vi "Extraction - Calculations.vi"(4 "Device":T1, 6 "Model":enum16{"pi", "tee"}(ring), 7 "2-port?":bool=TRUE, 8 "Freq for nominal C (MHz)":dbl=100.0, 9 "Y/Z-parameters":cdb[][](array[numeric]), 10 "Frequencies (Hz) in":dbl[](array[numeric]), 11 "S-parameters":cdb[][](array[numeric])) -> (0 "Heading":string[](array[string])=["Frequency (MHz)", "Capacitance (pF)", "Resistance (Ohm)", "Q", "Cshunt1 (pF)", "Cshunt2 (pF)", "SRF (MHz)"], 1 "index file values":dbl[](array[numeric]), 2 "index file heading":string[](array[string]), 3 "Frequency,C, R, Q/-IL, L, Cshunt1/2, Rshunt1/2, Lshunt1/2, SRF":dbl[][](array[numeric]), 5 "Graphs":T2)   [LabVIEW 2020]
panel:
  out "SRF (MHz)":dbl[](array[numeric])
  out "L":cluster{"Frequencies (Hz) in":dbl[], dbl[]}[](graph)
  out "S-para (mag)":dbl[][](array[numeric])
  out "Q":cluster{"Frequencies (Hz)":dbl[], dbl[]}(graph)
  out "R":cluster{"Frequencies (Hz)":dbl[], dbl[]}(graph)
  out "Capa":cluster{"Frequencies (Hz) in":dbl[], dbl[]}[](graph)
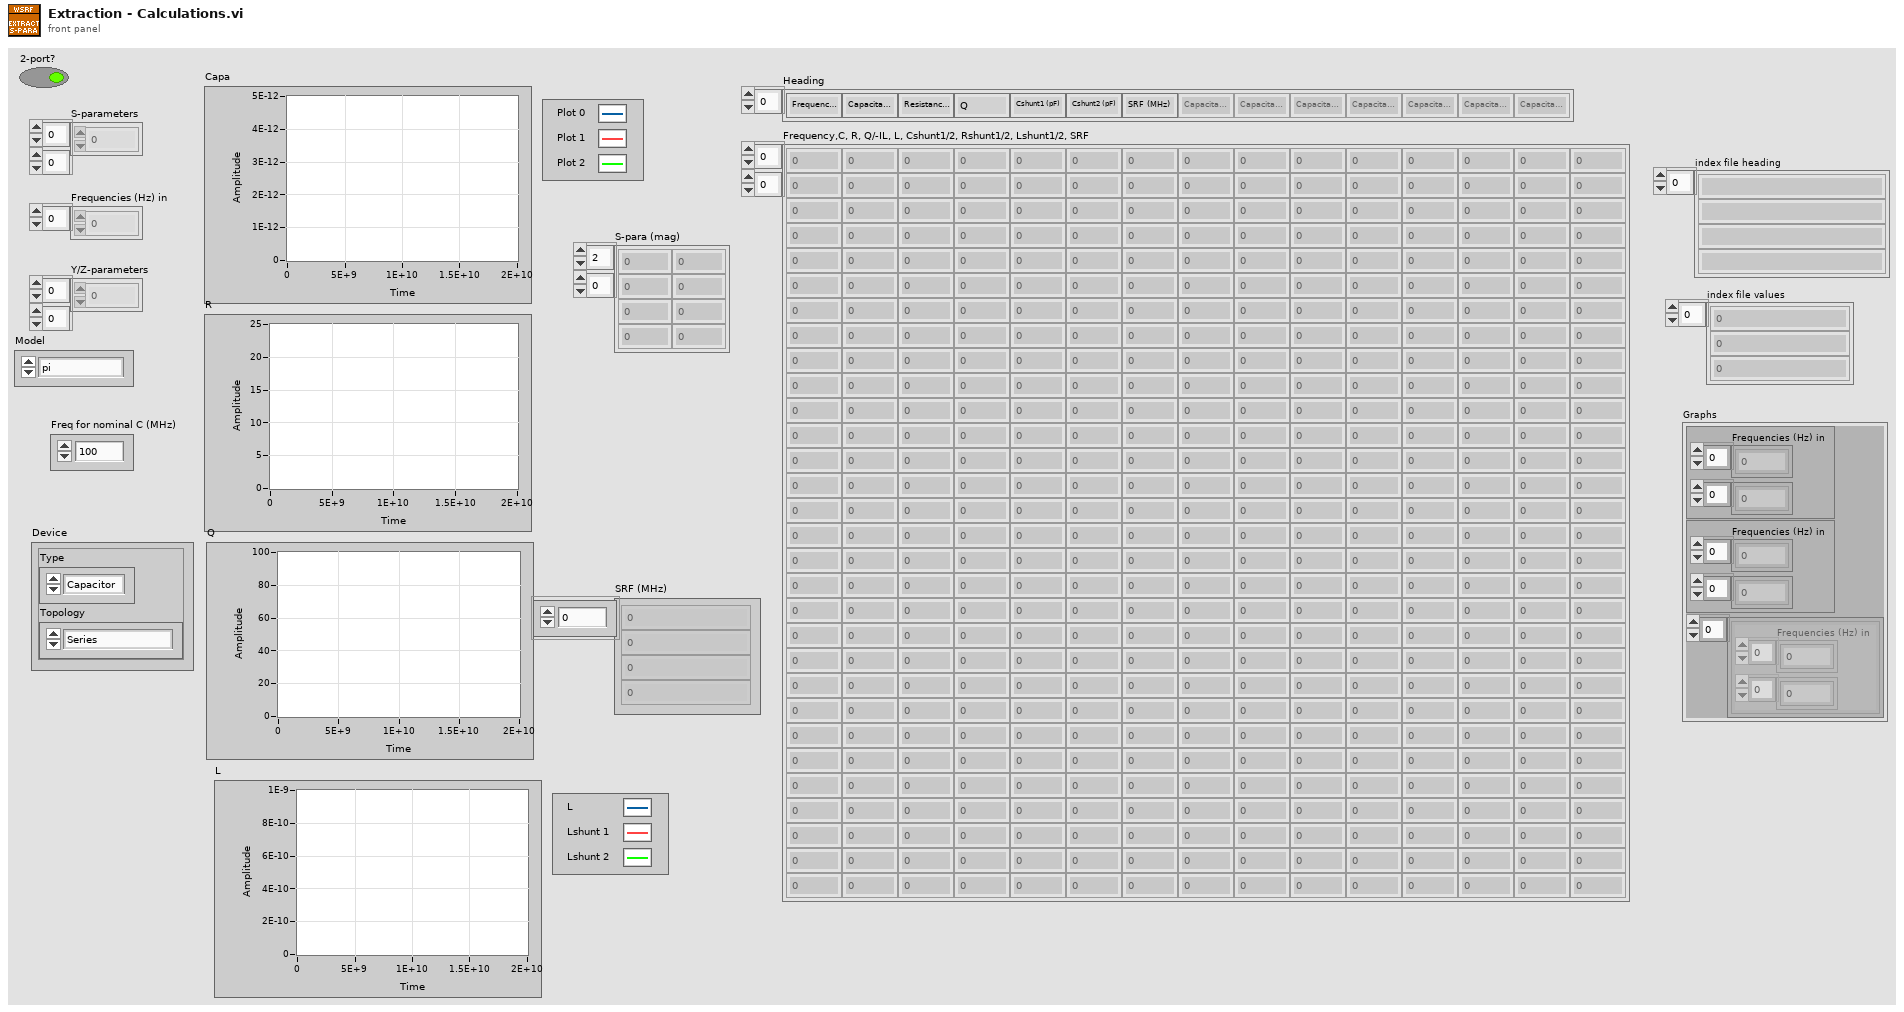
[diagram p1: front panel]
types:
  T1 = cluster{"Type":enum16{"Capacitor", "Switch"}, "Topology":enum16{"Series", "Parallel"}}
  T2 = cluster{cluster{"Frequencies (Hz) in":dbl[], dbl[]}, cluster{"Frequencies (Hz) in":dbl[], dbl[]}, cluster{"Frequencies (Hz) in":dbl[], dbl[]}[]}
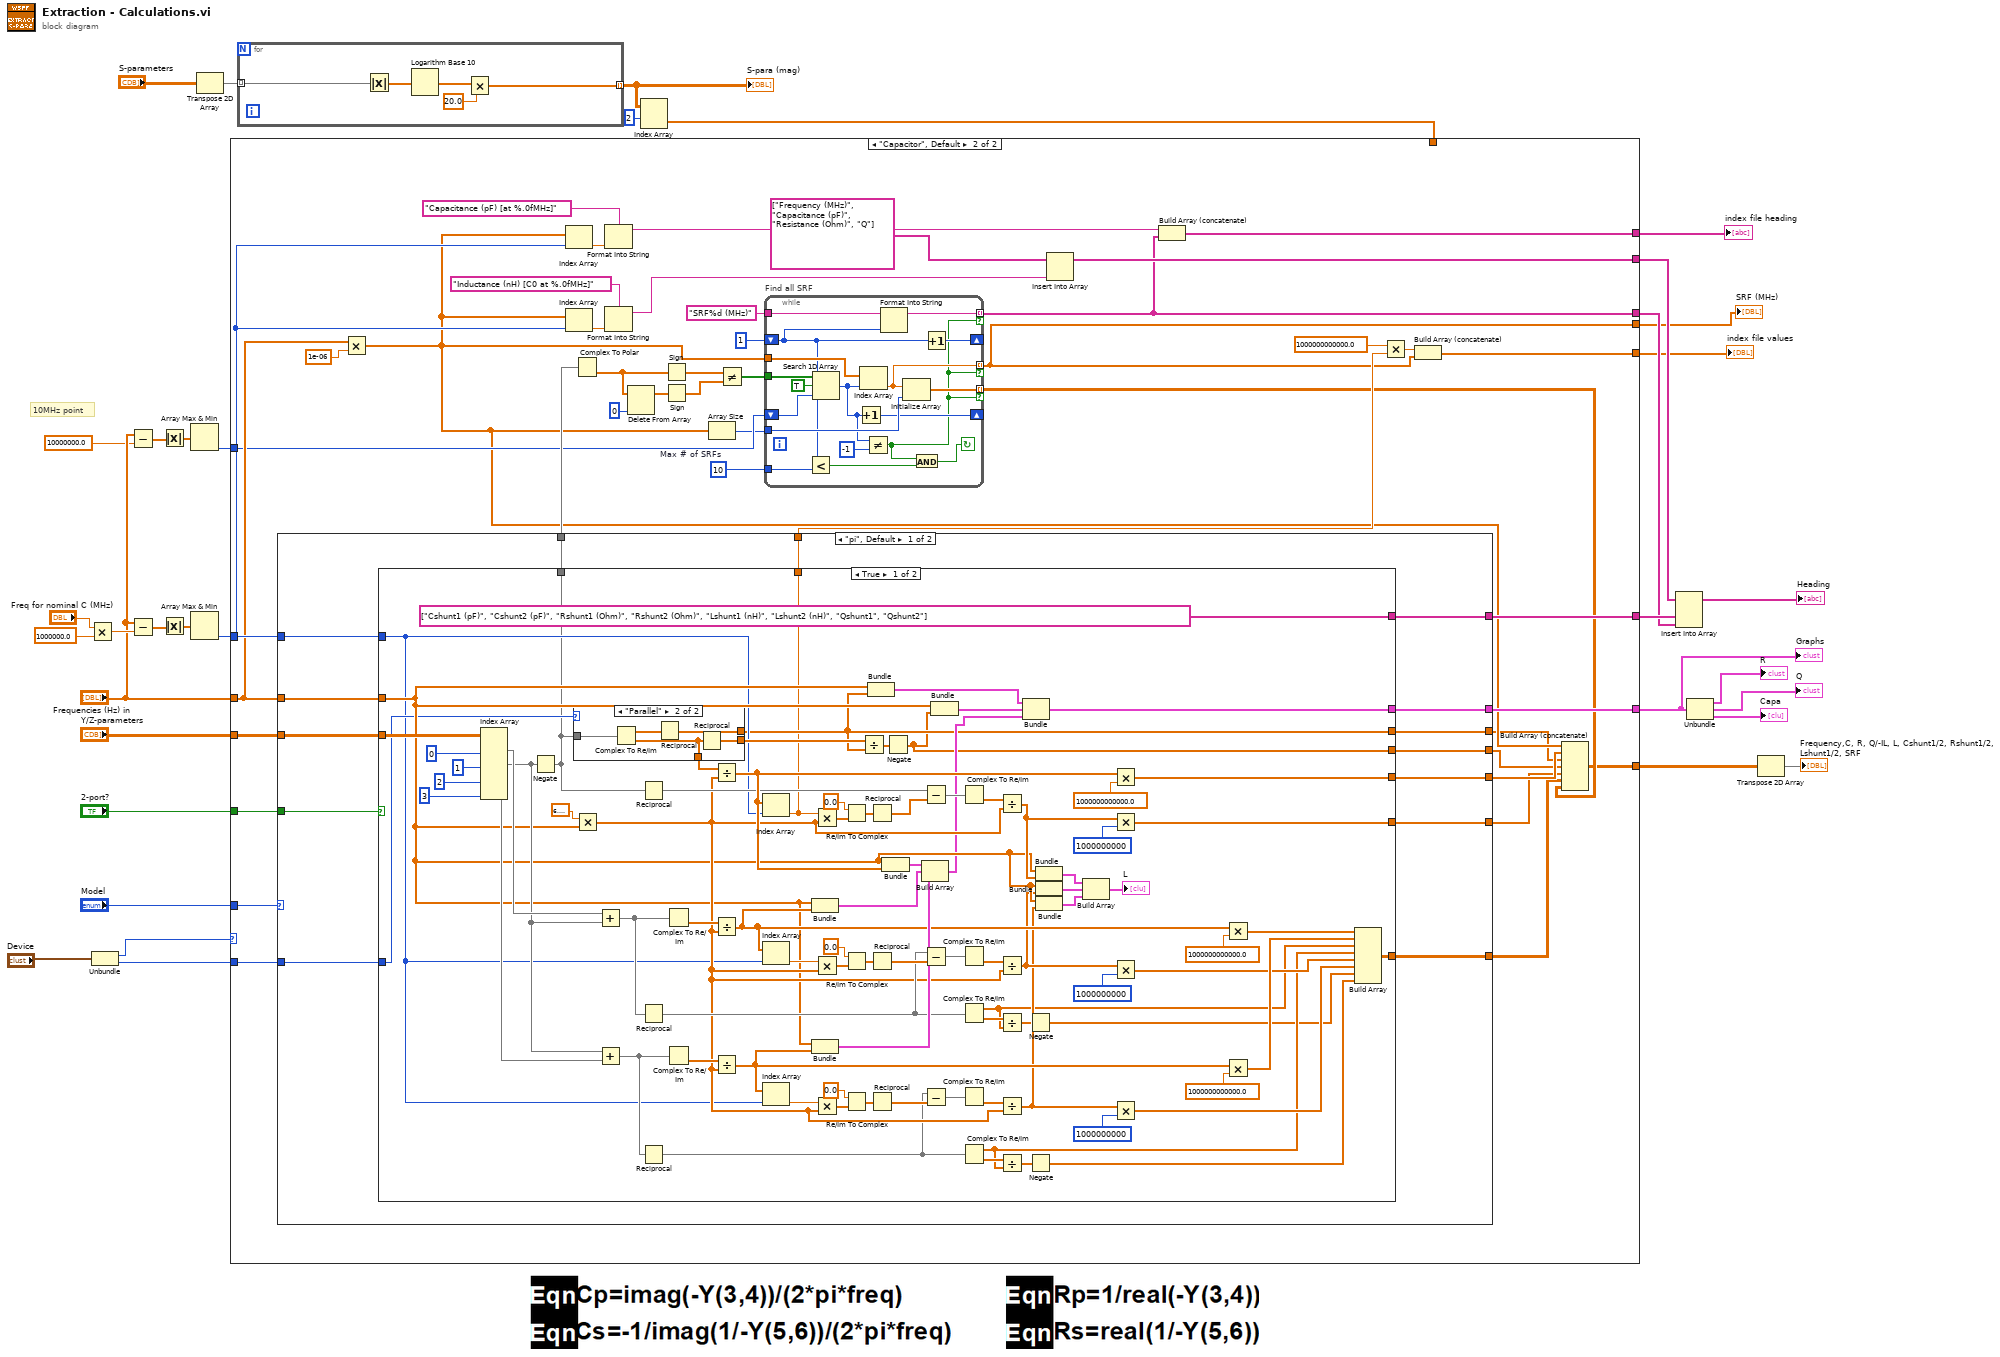
[diagram p0: block diagram]
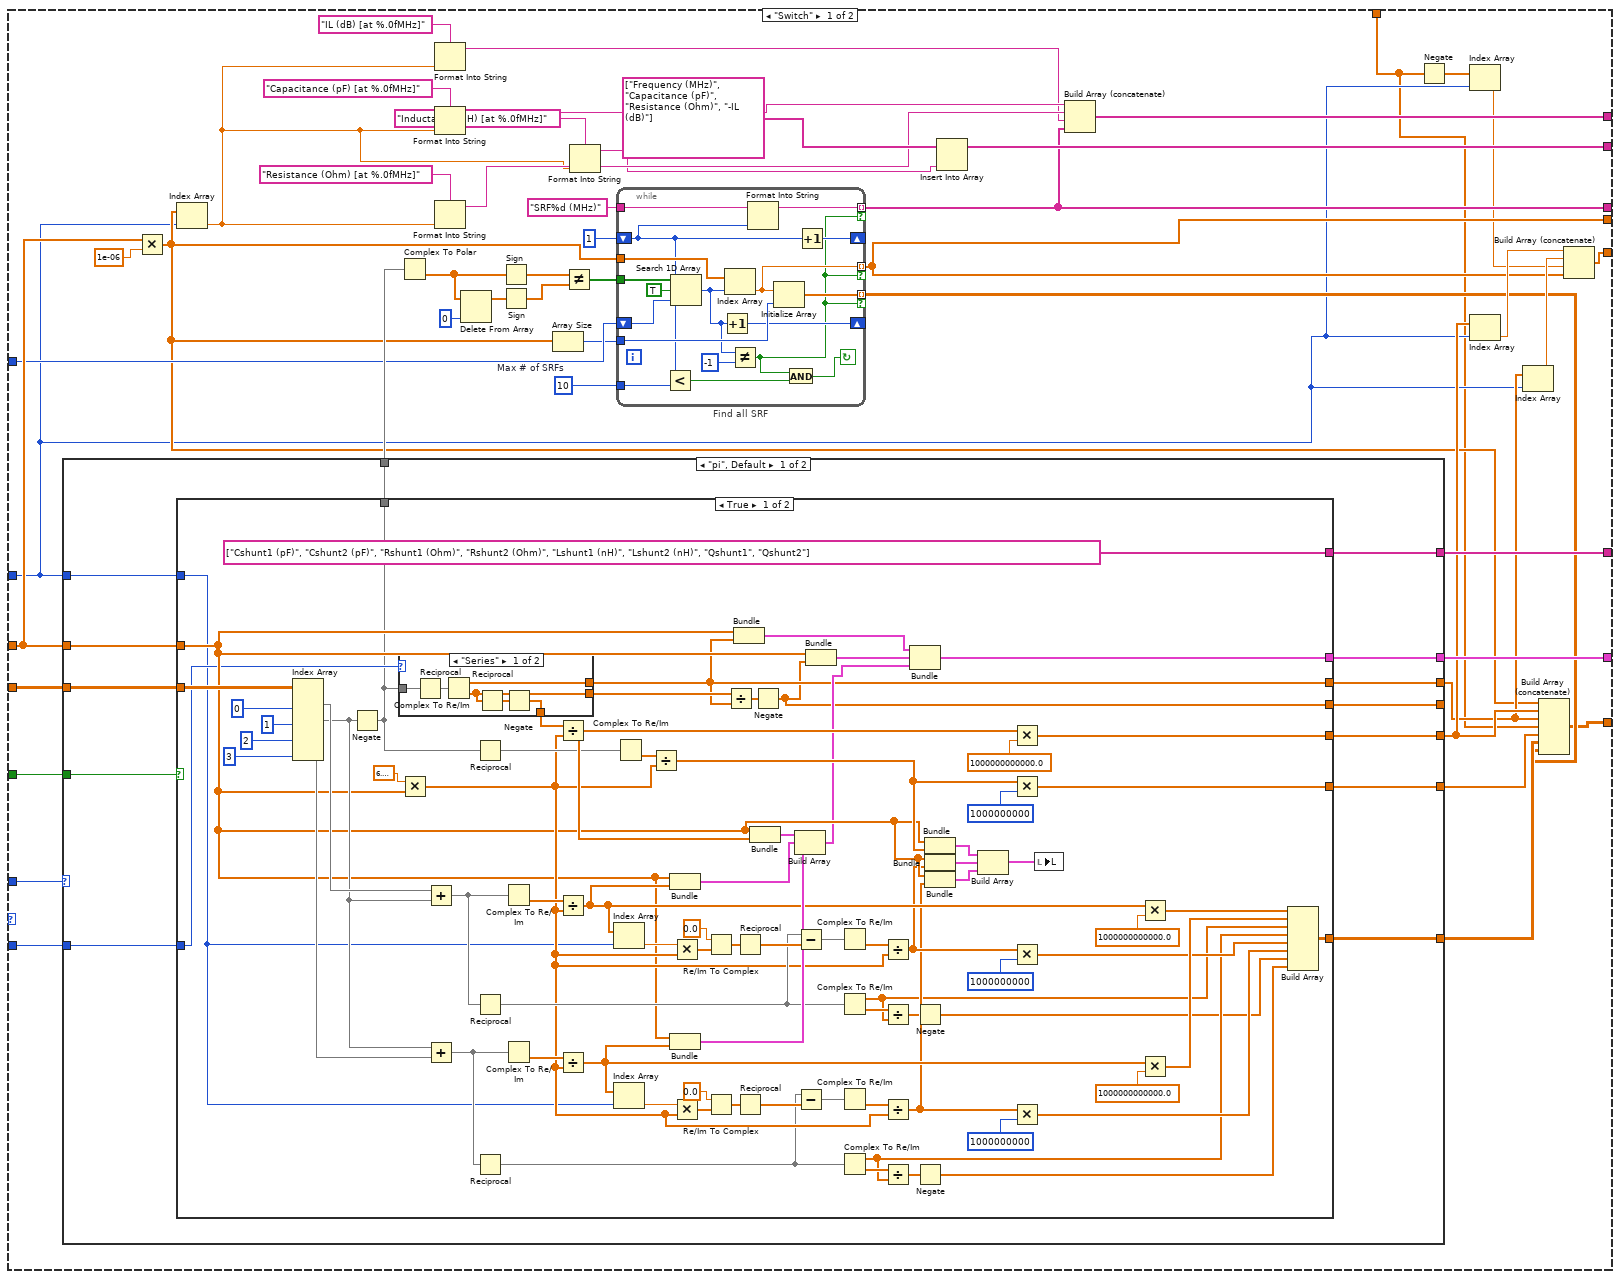
[diagram p2: hidden frame]
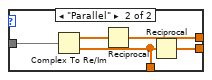
[diagram p3: hidden frame]
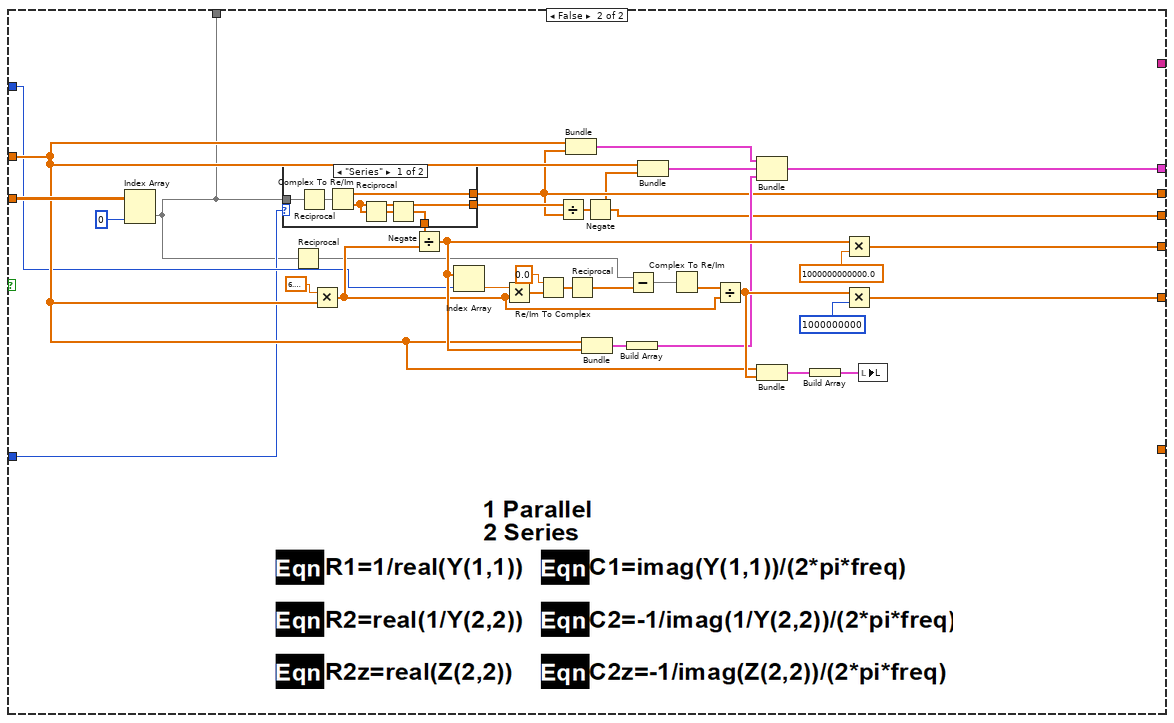
[diagram p4: hidden frame]
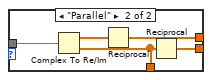
[diagram p5: hidden frame]
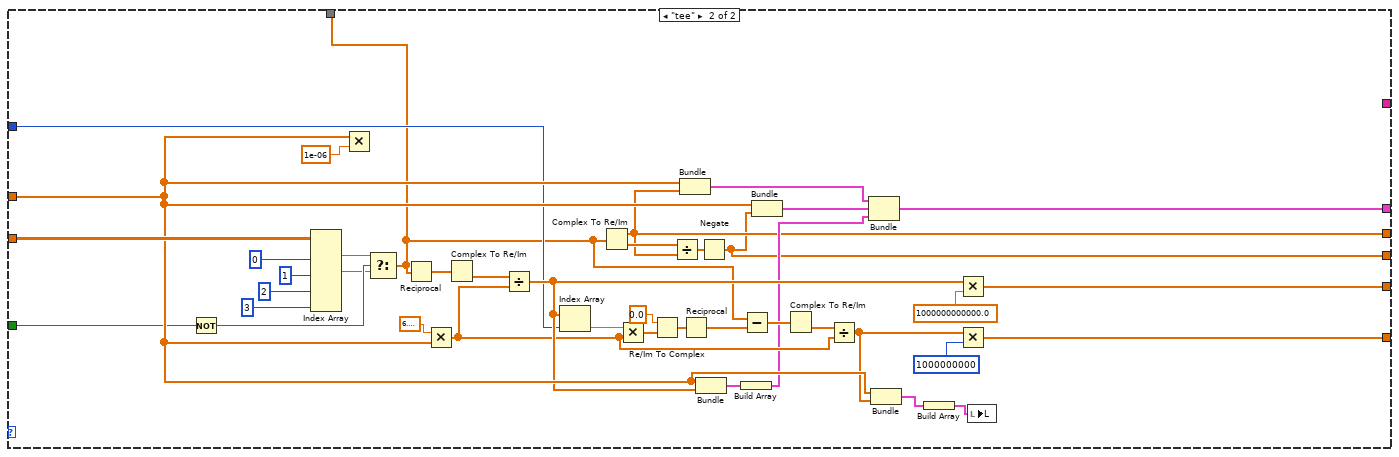
[diagram p6: hidden frame]
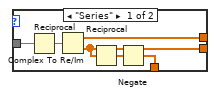
[diagram p7: hidden frame]
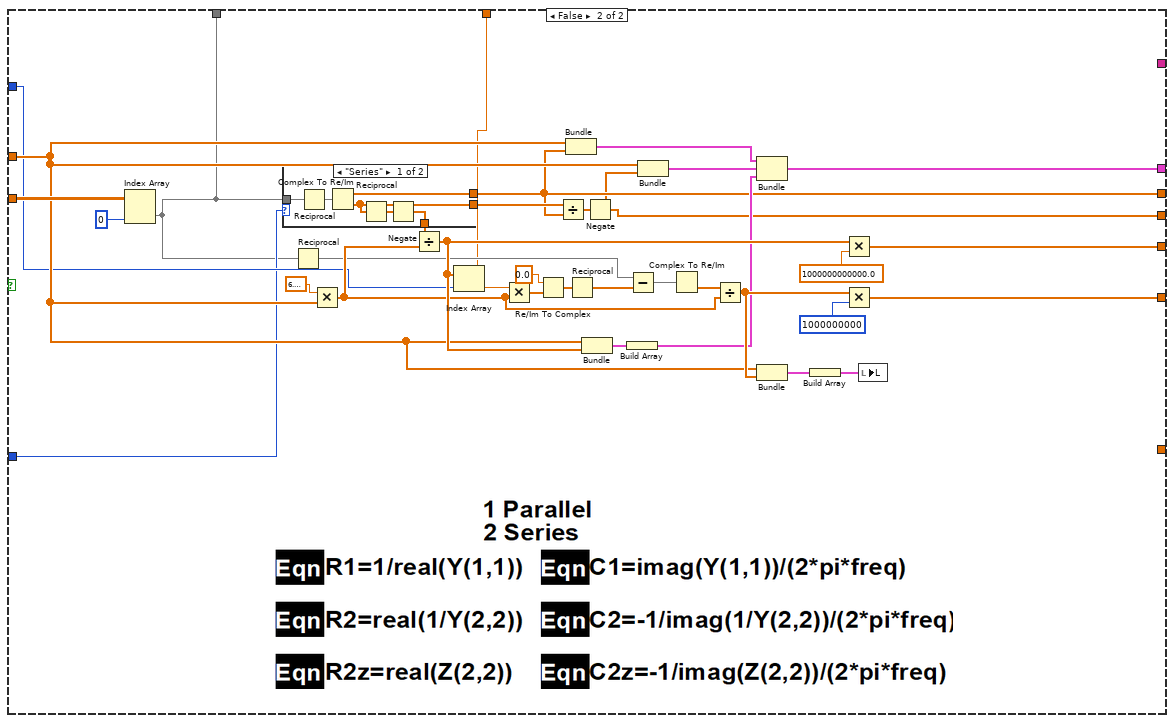
[diagram p8: hidden frame]
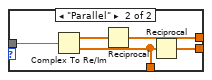
[diagram p9: hidden frame]
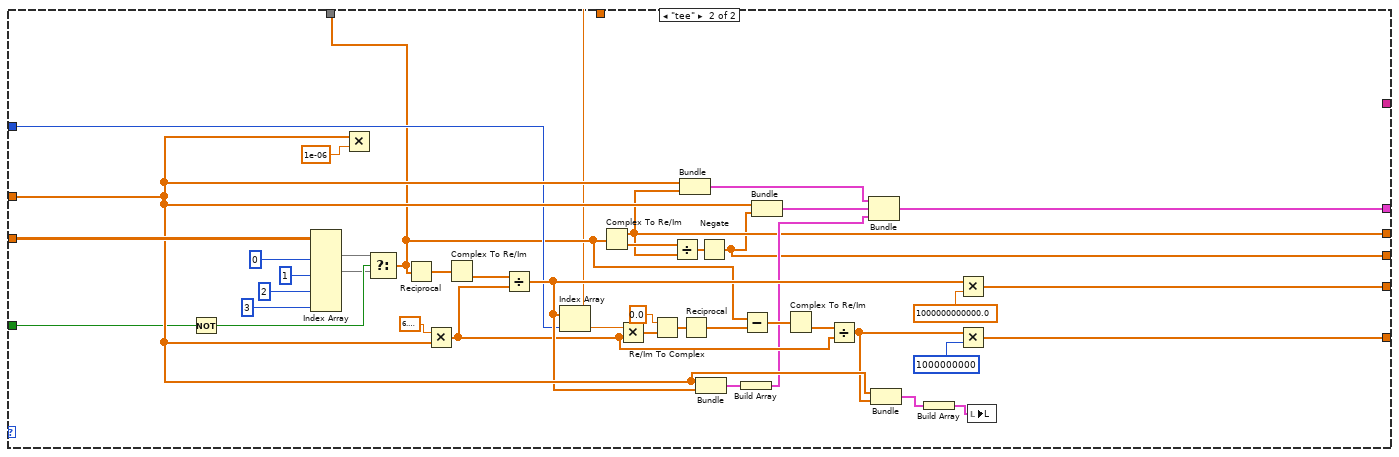
[diagram p10: hidden frame]
diagram:
  # "10MHz point"
  n1 = Multiply(x="Freq for nominal C (MHz)", y=1000000.0 ("Frequency (Hz)")) -> (x*y=w27:dbl)
  n2 = Unbundle("Device") -> ("Type"=w8:enum16{"Capacitor", "Switch"}, "Topology"=w9:enum16{"Series", "Parallel"})
  n3 = Subtract(x="Frequencies (Hz) in", y=10000000.0 ("Frequency (Hz)")) -> (x-y=w17:dbl[])
  n4 = Subtract(x="Frequencies (Hz) in", y=w27) -> (x-y=w26:dbl[])
  n5 = Absolute Value(x=w17) -> (abs(x)=w16:dbl[])
  n6 = Absolute Value(x=w26) -> (abs(x)=w25:dbl[])
  n7 = Array Max & Min(array=w16) -> (min index (indices)=w15:i32)  [unwired: 3 out]
  n8 = Array Max & Min(array=w25) -> (min index (indices)=w20:i32)  [unwired: 3 out]
  n9 = Transpose 2D Array(2D array="S-parameters") -> (transposed array=w32:cdb[][])
  n10 = for {
    tunnel: w32 -> [w37] mode=indexing
    tunnel: [w36] -> w3 mode=indexing
    n11 = Absolute Value(x=w37) -> (abs(x)=w38:dbl[])
    n12 = Logarithm Base 10(1:w38) -> (0:w39:dbl[])
    n13 = Multiply(x=w39, y=20.0) -> (x*y=w36:dbl[])
  }
  "S-para (mag)" <- w3
  n14 = Index Array(array=w3, index (row)=2) -> (element=w1:dbl[])  [unwired: 1 in]
  n15 = case shown="\"Capacitor\", Default" w8 {
    tunnel: "Y/Z-parameters" -> [w88 w340]
    tunnel: "2-port?" -> [w87 w339]
    tunnel: "Model" -> [w86 w338]
    tunnel: [w85 w337] -> w21
    tunnel: w20 -> [w47 w330]
    tunnel: "Frequencies (Hz) in" -> [w72 w317]
    tunnel: w15 -> [w71 w316]
    tunnel: [w67 w312] -> w13
    tunnel: [w66 w311] -> w12
    tunnel: [w65 w310] -> w11
    tunnel: w9 -> [w63 w308]
    tunnel: [w58 w307] -> w7
    tunnel: [w57 w306] -> w6
    tunnel: [w56 w305] -> w5
    tunnel: [w53 w298] -> w4
    tunnel: w1 -> [w42 _]
    frame "Switch" {
      w64 = 10  # Max # of SRFs
      n16 = case shown="\"pi\", Default" w86 {
        tunnel: w88 -> [w119 w296]
        tunnel: w72 -> [w114 w295]
        tunnel: w87 -> [w118 w294]
        tunnel: w47 -> [w115 w266]
        tunnel: w63 -> [w117 _]
        tunnel: [w116 w262] -> w85
        tunnel: [w110 w261] -> w74
        tunnel: [w107 w259] -> w61
        tunnel: [w113 w258] -> w51
        tunnel: [w112 w257] -> _
        tunnel: [w108 w256] -> w62
        tunnel: [w111 _] -> w55
        tunnel: [w109 _] -> w67
        frame "pi", Default {
          n17 = case shown="True" w118 {
            tunnel: [w198 _] -> w111
            tunnel: w119 -> [w193 w240]
            tunnel: w114 -> [w145 w226]
            tunnel: w115 -> [w122 w224]
            tunnel: w117 -> [w132 w223]
            tunnel: [w128 w217] -> w116
            tunnel: [w121 w216] -> w107
            tunnel: [w127 w215] -> w113
            tunnel: [w126 w214] -> w112
            tunnel: [w123 w213] -> w108
            tunnel: [w125 w211] -> w110
            tunnel: [string[] ["Cshunt1 (pF)", "Cshunt2 (pF)", "Rshunt1 (Ohm)", "Rshunt2 (Ohm)", "Lshunt1 (nH)", "Lshunt2 (nH)", "Qshunt1", "Qshunt2"] ("Heading") _] -> w109
            frame True {
              n18 = Index Array(array=w193, index (col) #1=0 ("disabled index (col)"), index (col) #2=1 ("disabled index (col)"), index (col) #3=2 ("index (col)"), index (col) #4=3 ("index (col)")) -> (element #1=w190:cdb[], element #2=w187:cdb[], element #4=w186:cdb[])  [unwired: 4 in, 1 out]
              n19 = Negate(x=w187) -> (-x=w125:cdb[])
              n20 = case shown="\"Series\"" w132 {
                tunnel: [w205 w208] -> w127
                tunnel: [w202 w207] -> w133
                tunnel: w125 -> [w204 w210]
                tunnel: [w200 w206] -> w134
                frame "Series" {
                  n21 = Reciprocal(x=w204) -> (1/x=w203:cdb[])
                  n22 = Complex To Re/Im(x + iy=w203) -> (x=w205:dbl[], y=w202:dbl[])
                  n23 = Reciprocal(x=w202) -> (1/x=w201:dbl[])
                  n24 = Negate(x=w201) -> (-x=w200:dbl[])
                }
                frame "Parallel" {
                  n25 = Complex To Re/Im(x + iy=w210) -> (x=w209:dbl[], y=w206:dbl[])
                  n26 = Reciprocal(x=w209) -> (1/x=w208:dbl[])
                  n27 = Reciprocal(x=w206) -> (1/x=w207:dbl[])
                }
              }
              n28 = Multiply(x=6.283185307179586, y=w145) -> (x*y=w155:dbl[])
              n29 = Add(x=w190, y=w187) -> (x+y=w175:cdb[])
              n30 = Add(x=w187, y=w186) -> (x+y=w174:cdb[])
              n31 = Reciprocal(x=w125) -> (1/x=w167:cdb[])
              n32 = Reciprocal(x=w175) -> (1/x=w156:cdb[])
              n33 = Reciprocal(x=w174) -> (1/x=w150:cdb[])
              n34 = Complex To Re/Im(x + iy=w175) -> (y=w189:dbl[])  [unwired: 1 out]
              n35 = Complex To Re/Im(x + iy=w174) -> (y=w188:dbl[])  [unwired: 1 out]
              n36 = Divide(x=w134, y=w155) -> (x/y=w178:dbl[])
              n37 = Divide(x=w189, y=w155) -> (x/y=w176:dbl[])
              n38 = Divide(x=w188, y=w155) -> (x/y=w177:dbl[])
              n39 = Index Array(array=w176, index=w122) -> (element=w173:dbl)
              n40 = Index Array(array=w177, index=w122) -> (element=w172:dbl)
              n41 = Complex To Re/Im(x + iy=w167) -> (y=w166:dbl[])  [unwired: 1 out]
              n42 = Divide(x=w166, y=w155) -> (x/y=w148:dbl[])
              n43 = Bundle("Frequencies (Hz) in"=w145, w176) -> (w182:cluster{"Frequencies (Hz) in":dbl[], dbl[]})  [unwired: 1 in]
              n44 = Bundle("Frequencies (Hz) in"=w145, w177) -> (w181:cluster{"Frequencies (Hz) in":dbl[], dbl[]})  [unwired: 1 in]
              n45 = Multiply(x=w173, y=w155) -> (x*y=w171:dbl[])
              n46 = Multiply(x=w172, y=w155) -> (x*y=w170:dbl[])
              n47 = Re/Im To Complex(1:w171, 2:0.0) -> (0:w161:cdb[])
              n48 = Re/Im To Complex(1:w170, 2:0.0) -> (0:w157:cdb[])
              n49 = Divide(x=w133, y=w127) -> (x/y=w197:dbl[])
              n50 = Bundle("Frequencies (Hz) in"=w145, w127) -> (w129:cluster{"Frequencies (Hz) in":dbl[], dbl[]})  [unwired: 1 in]
              n51 = Reciprocal(x=w161) -> (1/x=w162:cdb[])
              n52 = Reciprocal(x=w157) -> (1/x=w160:cdb[])
              n53 = Bundle("Frequencies (Hz) in"=w145, w178) -> (w180:cluster{"Frequencies (Hz) in":dbl[], dbl[]})  [unwired: 1 in]
              n54 = Negate(x=w197) -> (-x=w126:dbl[])
              n55 = Build Array(w180, w182, w181) -> (w131:cluster{"Frequencies (Hz) in":dbl[], dbl[]}[])
              n56 = Subtract(x=w156, y=w162) -> (x-y=w163:cdb[])
              n57 = Subtract(x=w150, y=w160) -> (x-y=w159:cdb[])
              n58 = Bundle("Frequencies (Hz) in"=w145, w126) -> (w130:cluster{"Frequencies (Hz) in":dbl[], dbl[]})  [unwired: 1 in]
              n59 = Complex To Re/Im(x + iy=w163) -> (y=w164:dbl[])  [unwired: 1 out]
              n60 = Complex To Re/Im(x + iy=w156) -> (x=w136:dbl[], y=w137:dbl[])
              n61 = Complex To Re/Im(x + iy=w159) -> (y=w158:dbl[])  [unwired: 1 out]
              n62 = Complex To Re/Im(x + iy=w150) -> (x=w141:dbl[], y=w142:dbl[])
              n63 = Divide(x=w164, y=w155) -> (x/y=w144:dbl[])
              n64 = Divide(x=w137, y=w136) -> (x/y=w138:dbl[])
              n65 = Divide(x=w158, y=w155) -> (x/y=w143:dbl[])
              n66 = Divide(x=w142, y=w141) -> (x/y=w140:dbl[])
              n67 = Bundle(w129, w130, w131) -> (w128:T2)  [unwired: 1 in]
              n68 = Negate(x=w138) -> (-x=w135:dbl[])
              n69 = Negate(x=w140) -> (-x=w139:dbl[])
              n70 = Bundle("Frequencies (Hz) in"=w145, w148) -> (w149:cluster{"Frequencies (Hz) in":dbl[], dbl[]})  [unwired: 1 in]
              n71 = Bundle("Frequencies (Hz) in"=w145, w144) -> (w147:cluster{"Frequencies (Hz) in":dbl[], dbl[]})  [unwired: 1 in]
              n72 = Bundle("Frequencies (Hz) in"=w145, w143) -> (w146:cluster{"Frequencies (Hz) in":dbl[], dbl[]})  [unwired: 1 in]
              n73 = Build Array(w149, w147, w146) -> (w120:cluster{"Frequencies (Hz) in":dbl[], dbl[]}[])
              n74 = Multiply(x=w178, y=1000000000000.0 ("Frequency (Hz)")) -> (x*y=w121:dbl[])
              n75 = Multiply(x=w148, y=1000000000 ("Frequency (Hz)")) -> (x*y=w123:dbl[])
              n76 = Multiply(x=w144, y=1000000000 ("Frequency (Hz)")) -> (x*y=w152:dbl[])
              n77 = Multiply(x=w143, y=1000000000 ("Frequency (Hz)")) -> (x*y=w151:dbl[])
              n78 = local write "L"(w120) -> ()
              n79 = Multiply(x=w176, y=1000000000000.0 ("Frequency (Hz)")) -> (x*y=w179:dbl[])
              n80 = Multiply(x=w177, y=1000000000000.0 ("Frequency (Hz)")) -> (x*y=w183:dbl[])
              n81 = Build Array(w179, w183, w136, w141, w152, w151, w135, w139) -> (w198:dbl[][])
            }
            frame False {
              n82 = Index Array(array=w240, index (col)=0 ("disabled index (col)")) -> (element=w211:cdb[])  [unwired: 1 in]
              n83 = case shown="\"Series\"" w223 {
                tunnel: [w250 w253] -> w215
                tunnel: [w247 w252] -> w243
                tunnel: w211 -> [w249 w255]
                tunnel: [w245 w251] -> w221
                frame "Series" {
                  n84 = Reciprocal(x=w249) -> (1/x=w248:cdb[])
                  n85 = Complex To Re/Im(x + iy=w248) -> (x=w250:dbl[], y=w247:dbl[])
                  n86 = Reciprocal(x=w247) -> (1/x=w246:dbl[])
                  n87 = Negate(x=w246) -> (-x=w245:dbl[])
                }
                frame "Parallel" {
                  n88 = Complex To Re/Im(x + iy=w255) -> (x=w254:dbl[], y=w251:dbl[])
                  n89 = Reciprocal(x=w254) -> (1/x=w253:dbl[])
                  n90 = Reciprocal(x=w251) -> (1/x=w252:dbl[])
                }
              }
              n91 = Reciprocal(x=w211) -> (1/x=w222:cdb[])
              n92 = Multiply(x=6.283185307179586, y=w226) -> (x*y=w229:dbl[])
              n93 = Divide(x=w221, y=w229) -> (x/y=w237:dbl[])
              n94 = Index Array(array=w237, index=w224) -> (element=w212:dbl)
              n95 = Multiply(x=w212, y=w229) -> (x*y=w236:dbl[])
              n96 = Re/Im To Complex(1:w236, 2:0.0) -> (0:w234:cdb[])
              n97 = Divide(x=w243, y=w215) -> (x/y=w244:dbl[])
              n98 = Bundle("Frequencies (Hz) in"=w226, w215) -> (w220:cluster{"Frequencies (Hz) in":dbl[], dbl[]})  [unwired: 1 in]
              n99 = Reciprocal(x=w234) -> (1/x=w233:cdb[])
              n100 = Bundle("Frequencies (Hz) in"=w226, w237) -> (w238:cluster{"Frequencies (Hz) in":dbl[], dbl[]})  [unwired: 1 in]
              n101 = Negate(x=w244) -> (-x=w214:dbl[])
              n102 = Build Array(w238) -> (w218:cluster{"Frequencies (Hz) in":dbl[], dbl[]}[])
              n103 = Subtract(x=w222, y=w233) -> (x-y=w232:cdb[])
              n104 = Bundle("Frequencies (Hz) in"=w226, w214) -> (w219:cluster{"Frequencies (Hz) in":dbl[], dbl[]})  [unwired: 1 in]
              n105 = Complex To Re/Im(x + iy=w232) -> (y=w231:dbl[])  [unwired: 1 out]
              n106 = Divide(x=w231, y=w229) -> (x/y=w227:dbl[])
              n107 = Bundle(w220, w219, w218) -> (w217:T2)  [unwired: 1 in]
              n108 = Bundle("Frequencies (Hz) in"=w226, w227) -> (w228:cluster{"Frequencies (Hz) in":dbl[], dbl[]})  [unwired: 1 in]
              n109 = Build Array(w228) -> (w225:cluster{"Frequencies (Hz) in":dbl[], dbl[]}[])
              n110 = Multiply(x=w237, y=1000000000000.0 ("Frequency (Hz)")) -> (x*y=w216:dbl[])
              n111 = Multiply(x=w227, y=1000000000 ("Frequency (Hz)")) -> (x*y=w213:dbl[])
              n112 = local write "L"(w225) -> ()
            }
          }
        }
        frame "tee" {
          n113 = Not(x=w294) -> (.not. x?=w269:bool)
          n114 = Index Array(array=w296, index (col) #1=0 ("disabled index (col)"), index (col) #2=1 ("disabled index (col)"), index (col) #3=2 ("index (col)"), index (col) #4=3 ("index (col)")) -> (element #1=w268:cdb[], element #2=w267:cdb[])  [unwired: 4 in, 2 out]
          n115 = Multiply(x=w295, y=1e-06 ("Frequency (Hz)")) -> ()  [unwired: 1 out]
          n116 = Select(t=w268, s=w269, f=w267) -> (s? t:f=w261:cdb[])
          n117 = Reciprocal(x=w261) -> (1/x=w270:cdb[])
          n118 = Multiply(x=6.283185307179586, y=w295) -> (x*y=w274:dbl[])
          n119 = Complex To Re/Im(x + iy=w270) -> (y=w287:dbl[])  [unwired: 1 out]
          n120 = Divide(x=w287, y=w274) -> (x/y=w282:dbl[])
          n121 = Index Array(array=w282, index=w266) -> (element=w260:dbl)
          n122 = Complex To Re/Im(x + iy=w261) -> (x=w258:dbl[], y=w291:dbl[])
          n123 = Multiply(x=w260, y=w274) -> (x*y=w281:dbl[])
          n124 = Re/Im To Complex(1:w281, 2:0.0) -> (0:w279:cdb[])
          n125 = Divide(x=w291, y=w258) -> (x/y=w292:dbl[])
          n126 = Bundle("Frequencies (Hz) in"=w295, w258) -> (w265:cluster{"Frequencies (Hz) in":dbl[], dbl[]})  [unwired: 1 in]
          n127 = Reciprocal(x=w279) -> (1/x=w278:cdb[])
          n128 = Bundle("Frequencies (Hz) in"=w295, w282) -> (w283:cluster{"Frequencies (Hz) in":dbl[], dbl[]})  [unwired: 1 in]
          n129 = Negate(x=w292) -> (-x=w257:dbl[])
          n130 = Build Array(w283) -> (w263:cluster{"Frequencies (Hz) in":dbl[], dbl[]}[])
          n131 = Subtract(x=w261, y=w278) -> (x-y=w277:cdb[])
          n132 = Bundle("Frequencies (Hz) in"=w295, w257) -> (w264:cluster{"Frequencies (Hz) in":dbl[], dbl[]})  [unwired: 1 in]
          n133 = Complex To Re/Im(x + iy=w277) -> (y=w276:dbl[])  [unwired: 1 out]
          n134 = Divide(x=w276, y=w274) -> (x/y=w272:dbl[])
          n135 = Bundle(w265, w264, w263) -> (w262:T2)  [unwired: 1 in]
          n136 = Bundle("Frequencies (Hz) in"=w295, w272) -> (w273:cluster{"Frequencies (Hz) in":dbl[], dbl[]})  [unwired: 1 in]
          n137 = Build Array(w273) -> (w271:cluster{"Frequencies (Hz) in":dbl[], dbl[]}[])
          n138 = Multiply(x=w282, y=1000000000000.0 ("Frequency (Hz)")) -> (x*y=w259:dbl[])
          n139 = Multiply(x=w272, y=1000000000 ("Frequency (Hz)")) -> (x*y=w256:dbl[])
          n140 = local write "L"(w271) -> ()
        }
      }
      n141 = Multiply(x=w72, y=1e-06 ("Frequency (Hz)")) -> (x*y=w49:dbl[])
      n142 = Index Array(array=w49, index=w47) -> (element=w43:dbl)
      n143 = Complex To Polar(r * e^(i*theta)=w74) -> (theta=w80:dbl[])  [unwired: 1 out]
      n144 = Format Into String(format string="IL (dB) [at %.0fMHz]", w43) -> (resulting string=w48:string)  [unwired: 2 in, 1 out]
      n145 = Format Into String(format string="Capacitance (pF) [at %.0fMHz]", w43) -> (resulting string=w83:string)  [unwired: 2 in, 1 out]
      n146 = Format Into String(format string="Resistance (Ohm) [at %.0fMHz]", w43) -> (resulting string=w52:string)  [unwired: 2 in, 1 out]
      n147 = Delete From Array(array=w80, index=0) -> (array with subset deleted=w78:dbl[])  [unwired: 1 in, 1 out]
      n148 = Sign(1:w80) -> (0:w77:dbl[])
      n149 = Sign(1:w78) -> (0:w76:dbl[])
      n150 = Array Size(array=w49) -> (size(s)=w70:i32)
      n151 = Not Equal?(x=w77, y=w76) -> (x != y?=w75:bool[])
      n152 = Format Into String(format string="Inductance (nH) [at %.0fMHz]", w43) -> (resulting string=w44:string)  [unwired: 2 in, 1 out]
      n153 = while "Find all SRF" {
        tunnel: w75 -> [w106]
        tunnel: w49 -> [w103]
        tunnel: [w101] -> w54 mode=indexing if=w91
        tunnel: w70 -> [w102]
        shift-right: [w100] -> _
        shift-left: w71 -> [w104]
        tunnel: [w99] -> w57 mode=indexing if=w91
        tunnel: "SRF%d (MHz)" ("element") -> [w96]
        tunnel: [w95] -> w65 mode=indexing if=w91
        shift-right: [w94] -> _
        shift-left: 1 -> [w93]
        tunnel: w64 -> [w89]
        stop <- w90 continue-if-true
        n154 = Less?(x=w93, y=w89) -> (x < y?=w92:bool)
        n155 = Search 1D Array(1D array=w106, element=TRUE, start index (0)=w104) -> (index of element=w98:i32)
        n156 = Increment(x=w98) -> (x+1=w100:i32)
        n157 = Index Array(array=w103, index=w98) -> (element=w99:dbl)
        n158 = Not Equal?(x=w98, y=-1) -> (x != y?=w91:bool)
        n159 = Format Into String(format string=w96, w93) -> (resulting string=w95:string)  [unwired: 2 in, 1 out]
        n160 = Initialize Array(w99, w102) -> (w101:dbl[])
        n161 = And(x=w91, y=w92) -> (x .and. y?=w90:bool)
        n162 = Increment(x=w93) -> (x+1=w94:i32)
      }
      n163 = Insert Into Array(array=string[] ["Frequency (MHz)", "Capacitance (pF)", "Resistance (Ohm)", "-IL (dB)"] ("Heading"), new element=w44) -> (w66:string[])  [unwired: 1 in]
      n164 = Build Array (concatenate)(w83, w52, w48, w65) -> (w56:string[])
      n165 = Negate(x=w42) -> (-x=w41:dbl[])
      n166 = Index Array(array=w41, index=w47) -> (element=w46:dbl)
      n167 = Index Array(array=w61, index=w47) -> (element=w59:dbl)
      n168 = Index Array(array=w51, index=w47) -> (element=w60:dbl)
      n169 = Build Array (concatenate)(w49, w61, w51, w42, w62, w55, w54) -> (w53:dbl[][])
      n170 = Build Array (concatenate)(w59, w60, w46, w57) -> (w58:dbl[])
    }
    frame "Capacitor", Default {
      w309 = 10  # Max # of SRFs
      n171 = case shown="\"pi\", Default" w338 {
        tunnel: w340 -> [w372 w555]
        tunnel: w317 -> [w367 w554]
        tunnel: w339 -> [w371 w553]
        tunnel: w330 -> [w368 w525]
        tunnel: w308 -> [w370 _]
        tunnel: [w369 w521] -> w337
        tunnel: [w360 w520] -> w320
        tunnel: [w361 w519] -> w319
        tunnel: [w366 w518] -> w303
        tunnel: [w365 w517] -> w302
        tunnel: [w364 w516] -> w297
        tunnel: [w363 w515] -> w301
        tunnel: [w362 _] -> w300
        tunnel: [w359 _] -> w312
        frame "pi", Default {
          n172 = case shown="True" w371 {
            tunnel: [w457 _] -> w362
            tunnel: w372 -> [w452 w499]
            tunnel: w367 -> [w398 w485]
            tunnel: w368 -> [w384 w483]
            tunnel: w370 -> [w385 w482]
            tunnel: [w380 w476] -> w369
            tunnel: [w378 w475] -> w366
            tunnel: [w377 w474] -> w365
            tunnel: [w376 w473] -> w364
            tunnel: [w379 w472] -> w363
            tunnel: [w375 w471] -> w361
            tunnel: [w374 w470] -> w360
            tunnel: [string[] ["Cshunt1 (pF)", "Cshunt2 (pF)", "Rshunt1 (Ohm)", "Rshunt2 (Ohm)", "Lshunt1 (nH)", "Lshunt2 (nH)", "Qshunt1", "Qshunt2"] ("Heading") _] -> w359
            frame True {
              n173 = Index Array(array=w452, index (col) #1=0 ("disabled index (col)"), index (col) #2=1 ("disabled index (col)"), index (col) #3=2 ("index (col)"), index (col) #4=3 ("index (col)")) -> (element #1=w449:cdb[], element #2=w446:cdb[], element #4=w445:cdb[])  [unwired: 4 in, 1 out]
              n174 = Negate(x=w446) -> (-x=w374:cdb[])
              n175 = case shown="\"Parallel\"" w385 {
                tunnel: [w464 w467] -> w377
                tunnel: [w461 w466] -> w386
                tunnel: w374 -> [w463 w469]
                tunnel: [w459 w465] -> w387
                frame "Series" {
                  n176 = Reciprocal(x=w463) -> (1/x=w462:cdb[])
                  n177 = Complex To Re/Im(x + iy=w462) -> (x=w464:dbl[], y=w461:dbl[])
                  n178 = Reciprocal(x=w461) -> (1/x=w460:dbl[])
                  n179 = Negate(x=w460) -> (-x=w459:dbl[])
                }
                frame "Parallel" {
                  n180 = Complex To Re/Im(x + iy=w469) -> (x=w468:dbl[], y=w465:dbl[])
                  n181 = Reciprocal(x=w468) -> (1/x=w467:dbl[])
                  n182 = Reciprocal(x=w465) -> (1/x=w466:dbl[])
                }
              }
              n183 = Multiply(x=6.283185307179586, y=w398) -> (x*y=w409:dbl[])
              n184 = Add(x=w449, y=w446) -> (x+y=w434:cdb[])
              n185 = Add(x=w446, y=w445) -> (x+y=w433:cdb[])
              n186 = Reciprocal(x=w374) -> (1/x=w423:cdb[])
              n187 = Reciprocal(x=w434) -> (1/x=w410:cdb[])
              n188 = Reciprocal(x=w433) -> (1/x=w404:cdb[])
              n189 = Complex To Re/Im(x + iy=w434) -> (y=w448:dbl[])  [unwired: 1 out]
              n190 = Complex To Re/Im(x + iy=w433) -> (y=w447:dbl[])  [unwired: 1 out]
              n191 = Divide(x=w387, y=w409) -> (x/y=w437:dbl[])
              n192 = Divide(x=w448, y=w409) -> (x/y=w435:dbl[])
              n193 = Divide(x=w447, y=w409) -> (x/y=w436:dbl[])
              n194 = Index Array(array=w437, index=w384) -> (element=w375:dbl)
              n195 = Index Array(array=w435, index=w384) -> (element=w432:dbl)
              n196 = Index Array(array=w436, index=w384) -> (element=w431:dbl)
              n197 = Bundle("Frequencies (Hz) in"=w398, w435) -> (w441:cluster{"Frequencies (Hz) in":dbl[], dbl[]})  [unwired: 1 in]
              n198 = Bundle("Frequencies (Hz) in"=w398, w436) -> (w440:cluster{"Frequencies (Hz) in":dbl[], dbl[]})  [unwired: 1 in]
              n199 = Multiply(x=w375, y=w409) -> (x*y=w430:dbl[])
              n200 = Multiply(x=w432, y=w409) -> (x*y=w429:dbl[])
              n201 = Multiply(x=w431, y=w409) -> (x*y=w428:dbl[])
              n202 = Re/Im To Complex(1:w430, 2:0.0) -> (0:w424:cdb[])
              n203 = Re/Im To Complex(1:w429, 2:0.0) -> (0:w415:cdb[])
              n204 = Re/Im To Complex(1:w428, 2:0.0) -> (0:w411:cdb[])
              n205 = Divide(x=w386, y=w377) -> (x/y=w456:dbl[])
              n206 = Bundle("Frequencies (Hz) in"=w398, w377) -> (w381:cluster{"Frequencies (Hz) in":dbl[], dbl[]})  [unwired: 1 in]
              n207 = Reciprocal(x=w424) -> (1/x=w422:cdb[])
              n208 = Reciprocal(x=w415) -> (1/x=w416:cdb[])
              n209 = Reciprocal(x=w411) -> (1/x=w414:cdb[])
              n210 = Bundle("Frequencies (Hz) in"=w398, w437) -> (w439:cluster{"Frequencies (Hz) in":dbl[], dbl[]})  [unwired: 1 in]
              n211 = Negate(x=w456) -> (-x=w376:dbl[])
              n212 = Build Array(w439, w441, w440) -> (w383:cluster{"Frequencies (Hz) in":dbl[], dbl[]}[])
              n213 = Subtract(x=w423, y=w422) -> (x-y=w421:cdb[])
              n214 = Subtract(x=w410, y=w416) -> (x-y=w417:cdb[])
              n215 = Subtract(x=w404, y=w414) -> (x-y=w413:cdb[])
              n216 = Bundle("Frequencies (Hz) in"=w398, w376) -> (w382:cluster{"Frequencies (Hz) in":dbl[], dbl[]})  [unwired: 1 in]
              n217 = Complex To Re/Im(x + iy=w421) -> (y=w420:dbl[])  [unwired: 1 out]
              n218 = Complex To Re/Im(x + iy=w417) -> (y=w418:dbl[])  [unwired: 1 out]
              n219 = Complex To Re/Im(x + iy=w410) -> (x=w389:dbl[], y=w390:dbl[])
              n220 = Complex To Re/Im(x + iy=w413) -> (y=w412:dbl[])  [unwired: 1 out]
              n221 = Complex To Re/Im(x + iy=w404) -> (x=w394:dbl[], y=w395:dbl[])
              n222 = Divide(x=w420, y=w409) -> (x/y=w401:dbl[])
              n223 = Divide(x=w418, y=w409) -> (x/y=w397:dbl[])
              n224 = Divide(x=w390, y=w389) -> (x/y=w391:dbl[])
              n225 = Divide(x=w412, y=w409) -> (x/y=w396:dbl[])
              n226 = Divide(x=w395, y=w394) -> (x/y=w393:dbl[])
              n227 = Bundle(w381, w382, w383) -> (w380:T2)  [unwired: 1 in]
              n228 = Negate(x=w391) -> (-x=w388:dbl[])
              n229 = Negate(x=w393) -> (-x=w392:dbl[])
              n230 = Bundle("Frequencies (Hz) in"=w398, w401) -> (w402:cluster{"Frequencies (Hz) in":dbl[], dbl[]})  [unwired: 1 in]
              n231 = Bundle("Frequencies (Hz) in"=w398, w397) -> (w400:cluster{"Frequencies (Hz) in":dbl[], dbl[]})  [unwired: 1 in]
              n232 = Bundle("Frequencies (Hz) in"=w398, w396) -> (w399:cluster{"Frequencies (Hz) in":dbl[], dbl[]})  [unwired: 1 in]
              n233 = Build Array(w402, w400, w399) -> (→"L":cluster{"Frequencies (Hz) in":dbl[], dbl[]}[])
              n234 = Multiply(x=w437, y=1000000000000.0 ("Frequency (Hz)")) -> (x*y=w378:dbl[])
              n235 = Multiply(x=w401, y=1000000000 ("Frequency (Hz)")) -> (x*y=w379:dbl[])
              n236 = Multiply(x=w397, y=1000000000 ("Frequency (Hz)")) -> (x*y=w406:dbl[])
              n237 = Multiply(x=w396, y=1000000000 ("Frequency (Hz)")) -> (x*y=w405:dbl[])
              n238 = Multiply(x=w435, y=1000000000000.0 ("Frequency (Hz)")) -> (x*y=w438:dbl[])
              n239 = Multiply(x=w436, y=1000000000000.0 ("Frequency (Hz)")) -> (x*y=w442:dbl[])
              n240 = Build Array(w438, w442, w389, w394, w406, w405, w388, w392) -> (w457:dbl[][])
            }
            frame False {
              n241 = Index Array(array=w499, index (col)=0 ("disabled index (col)")) -> (element=w470:cdb[])  [unwired: 1 in]
              n242 = case shown="\"Series\"" w482 {
                tunnel: [w509 w512] -> w474
                tunnel: [w506 w511] -> w502
                tunnel: w470 -> [w508 w514]
                tunnel: [w504 w510] -> w480
                frame "Series" {
                  n243 = Reciprocal(x=w508) -> (1/x=w507:cdb[])
                  n244 = Complex To Re/Im(x + iy=w507) -> (x=w509:dbl[], y=w506:dbl[])
                  n245 = Reciprocal(x=w506) -> (1/x=w505:dbl[])
                  n246 = Negate(x=w505) -> (-x=w504:dbl[])
                }
                frame "Parallel" {
                  n247 = Complex To Re/Im(x + iy=w514) -> (x=w513:dbl[], y=w510:dbl[])
                  n248 = Reciprocal(x=w513) -> (1/x=w512:dbl[])
                  n249 = Reciprocal(x=w510) -> (1/x=w511:dbl[])
                }
              }
              n250 = Reciprocal(x=w470) -> (1/x=w481:cdb[])
              n251 = Multiply(x=6.283185307179586, y=w485) -> (x*y=w488:dbl[])
              n252 = Divide(x=w480, y=w488) -> (x/y=w496:dbl[])
              n253 = Index Array(array=w496, index=w483) -> (element=w471:dbl)
              n254 = Multiply(x=w471, y=w488) -> (x*y=w495:dbl[])
              n255 = Re/Im To Complex(1:w495, 2:0.0) -> (0:w493:cdb[])
              n256 = Divide(x=w502, y=w474) -> (x/y=w503:dbl[])
              n257 = Bundle("Frequencies (Hz) in"=w485, w474) -> (w479:cluster{"Frequencies (Hz) in":dbl[], dbl[]})  [unwired: 1 in]
              n258 = Reciprocal(x=w493) -> (1/x=w492:cdb[])
              n259 = Bundle("Frequencies (Hz) in"=w485, w496) -> (w497:cluster{"Frequencies (Hz) in":dbl[], dbl[]})  [unwired: 1 in]
              n260 = Negate(x=w503) -> (-x=w473:dbl[])
              n261 = Build Array(w497) -> (w477:cluster{"Frequencies (Hz) in":dbl[], dbl[]}[])
              n262 = Subtract(x=w481, y=w492) -> (x-y=w491:cdb[])
              n263 = Bundle("Frequencies (Hz) in"=w485, w473) -> (w478:cluster{"Frequencies (Hz) in":dbl[], dbl[]})  [unwired: 1 in]
              n264 = Complex To Re/Im(x + iy=w491) -> (y=w490:dbl[])  [unwired: 1 out]
              n265 = Divide(x=w490, y=w488) -> (x/y=w486:dbl[])
              n266 = Bundle(w479, w478, w477) -> (w476:T2)  [unwired: 1 in]
              n267 = Bundle("Frequencies (Hz) in"=w485, w486) -> (w487:cluster{"Frequencies (Hz) in":dbl[], dbl[]})  [unwired: 1 in]
              n268 = Build Array(w487) -> (w484:cluster{"Frequencies (Hz) in":dbl[], dbl[]}[])
              n269 = Multiply(x=w496, y=1000000000000.0 ("Frequency (Hz)")) -> (x*y=w475:dbl[])
              n270 = Multiply(x=w486, y=1000000000 ("Frequency (Hz)")) -> (x*y=w472:dbl[])
              n271 = local write "L"(w484) -> ()
            }
          }
        }
        frame "tee" {
          n272 = Not(x=w553) -> (.not. x?=w528:bool)
          n273 = Index Array(array=w555, index (col) #1=0 ("disabled index (col)"), index (col) #2=1 ("disabled index (col)"), index (col) #3=2 ("index (col)"), index (col) #4=3 ("index (col)")) -> (element #1=w527:cdb[], element #2=w526:cdb[])  [unwired: 4 in, 2 out]
          n274 = Multiply(x=w554, y=1e-06 ("Frequency (Hz)")) -> ()  [unwired: 1 out]
          n275 = Select(t=w527, s=w528, f=w526) -> (s? t:f=w520:cdb[])
          n276 = Reciprocal(x=w520) -> (1/x=w529:cdb[])
          n277 = Multiply(x=6.283185307179586, y=w554) -> (x*y=w533:dbl[])
          n278 = Complex To Re/Im(x + iy=w529) -> (y=w546:dbl[])  [unwired: 1 out]
          n279 = Divide(x=w546, y=w533) -> (x/y=w541:dbl[])
          n280 = Index Array(array=w541, index=w525) -> (element=w519:dbl)
          n281 = Complex To Re/Im(x + iy=w520) -> (x=w517:dbl[], y=w550:dbl[])
          n282 = Multiply(x=w519, y=w533) -> (x*y=w540:dbl[])
          n283 = Re/Im To Complex(1:w540, 2:0.0) -> (0:w538:cdb[])
          n284 = Divide(x=w550, y=w517) -> (x/y=w551:dbl[])
          n285 = Bundle("Frequencies (Hz) in"=w554, w517) -> (w524:cluster{"Frequencies (Hz) in":dbl[], dbl[]})  [unwired: 1 in]
          n286 = Reciprocal(x=w538) -> (1/x=w537:cdb[])
          n287 = Bundle("Frequencies (Hz) in"=w554, w541) -> (w542:cluster{"Frequencies (Hz) in":dbl[], dbl[]})  [unwired: 1 in]
          n288 = Negate(x=w551) -> (-x=w516:dbl[])
          n289 = Build Array(w542) -> (w522:cluster{"Frequencies (Hz) in":dbl[], dbl[]}[])
          n290 = Subtract(x=w520, y=w537) -> (x-y=w536:cdb[])
          n291 = Bundle("Frequencies (Hz) in"=w554, w516) -> (w523:cluster{"Frequencies (Hz) in":dbl[], dbl[]})  [unwired: 1 in]
          n292 = Complex To Re/Im(x + iy=w536) -> (y=w535:dbl[])  [unwired: 1 out]
          n293 = Divide(x=w535, y=w533) -> (x/y=w531:dbl[])
          n294 = Bundle(w524, w523, w522) -> (w521:T2)  [unwired: 1 in]
          n295 = Bundle("Frequencies (Hz) in"=w554, w531) -> (w532:cluster{"Frequencies (Hz) in":dbl[], dbl[]})  [unwired: 1 in]
          n296 = Build Array(w532) -> (w530:cluster{"Frequencies (Hz) in":dbl[], dbl[]}[])
          n297 = Multiply(x=w541, y=1000000000000.0 ("Frequency (Hz)")) -> (x*y=w518:dbl[])
          n298 = Multiply(x=w531, y=1000000000 ("Frequency (Hz)")) -> (x*y=w515:dbl[])
          n299 = local write "L"(w530) -> ()
        }
      }
      n300 = Multiply(x=w317, y=1e-06 ("Frequency (Hz)")) -> (x*y=w304:dbl[])
      n301 = Index Array(array=w304, index=w330) -> (element=w336:dbl)
      n302 = Index Array(array=w304, index=w330) -> (element=w331:dbl)
      n303 = Complex To Polar(r * e^(i*theta)=w320) -> (theta=w328:dbl[])  [unwired: 1 out]
      n304 = Format Into String(format string="Capacitance (pF) [at %.0fMHz]", w336) -> (resulting string=w334:string)  [unwired: 2 in, 1 out]
      n305 = Format Into String(format string="Inductance (nH) [C0 at %.0fMHz]", w331) -> (resulting string=w332:string)  [unwired: 2 in, 1 out]
      n306 = Delete From Array(array=w328, index=0) -> (array with subset deleted=w326:dbl[])  [unwired: 1 in, 1 out]
      n307 = Sign(1:w328) -> (0:w325:dbl[])
      n308 = Sign(1:w326) -> (0:w324:dbl[])
      n309 = Array Size(array=w304) -> (size(s)=w315:i32)
      n310 = Not Equal?(x=w325, y=w324) -> (x != y?=w323:bool[])
      n311 = while "Find all SRF" {
        tunnel: w323 -> [w358]
        tunnel: w304 -> [w355]
        tunnel: [w353] -> w299 mode=indexing if=w343
        tunnel: w315 -> [w354]
        shift-right: [w352] -> _
        shift-left: w316 -> [w356]
        tunnel: [w351] -> w306 mode=indexing if=w343
        tunnel: "SRF%d (MHz)" ("element") -> [w348]
        tunnel: [w347] -> w310 mode=indexing if=w343
        shift-right: [w346] -> _
        shift-left: 1 -> [w345]
        tunnel: w309 -> [w341]
        stop <- w342 continue-if-true
        n312 = Less?(x=w345, y=w341) -> (x < y?=w344:bool)
        n313 = Search 1D Array(1D array=w358, element=TRUE, start index (0)=w356) -> (index of element=w350:i32)
        n314 = Increment(x=w350) -> (x+1=w352:i32)
        n315 = Index Array(array=w355, index=w350) -> (element=w351:dbl)
        n316 = Not Equal?(x=w350, y=-1) -> (x != y?=w343:bool)
        n317 = Format Into String(format string=w348, w345) -> (resulting string=w347:string)  [unwired: 2 in, 1 out]
        n318 = Initialize Array(w351, w354) -> (w353:dbl[])
        n319 = And(x=w343, y=w344) -> (x .and. y?=w342:bool)
        n320 = Increment(x=w345) -> (x+1=w346:i32)
      }
      n321 = Insert Into Array(array=string[] ["Frequency (MHz)", "Capacitance (pF)", "Resistance (Ohm)", "Q"] ("Heading"), new element=w332) -> (w311:string[])  [unwired: 1 in]
      n322 = Build Array (concatenate)(w334, w310) -> (w305:string[])
      n323 = Multiply(x=1000000000000.0 ("Frequency (Hz)"), y=w319) -> (x*y=w321:dbl)
      n324 = Build Array (concatenate)(w321, w306) -> (w307:dbl[])
      n325 = Build Array (concatenate)(w304, w303, w302, w297, w301, w300, w299) -> (w298:dbl[][])
    }
  }
  "Graphs" <- w21
  "index file values" <- w7
  "SRF (MHz)" <- w6
  "index file heading" <- w5
  n326 = Insert Into Array(array=w12, new element #1=w13, new element #2=w11) -> (→"Heading":string[])  [unwired: 1 in]
  n327 = Unbundle(w21) -> (→"R":cluster{"Frequencies (Hz) in":dbl[], dbl[]}, →"Q":cluster{"Frequencies (Hz) in":dbl[], dbl[]}, →"Capa":cluster{"Frequencies (Hz) in":dbl[], dbl[]}[])
  n328 = Transpose 2D Array(2D array=w4) -> (transposed array=→"Frequency,C, R, Q/-IL, L, Cshunt1/2, Rshunt1/2, Lshunt1/2, SRF":dbl[][])
